vi "Write Hardware Handles.vi"(8 "error in":errorcluster, 10 "hardware handles":T1, 11 "Shared Resources in":refnum<class "Shared Resources.lvclass">) -> (0 "error out":errorcluster, 3 "Shared Resources out":refnum<class "Shared Resources.lvclass">)   [LabVIEW 2020, in "Ballard MIL-STD-1553 Engine.lvlib" / "Implementation.lvlib" / "Shared Resources.lvclass"]
uses:
  Shared Resources.lvclass
  Custom Device/Hardware Handles.ctl
  Shared Resources.lvclass/Shared Resources.ctl
  Custom Device/Custom Device.lvlib
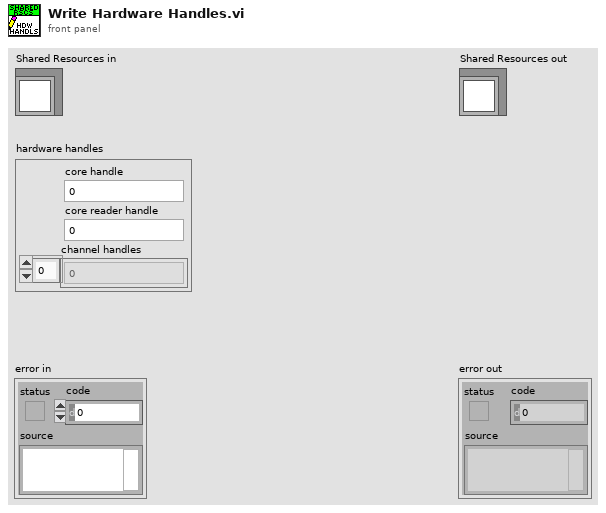
[diagram p1: front panel]
types:
  T1 = typedef "Ballard MIL-STD-1553 Engine.lvlib/Custom Device.lvlib/Hardware Handles.ctl" = cluster{"core handle":u64, "core reader handle":u64, "channel handles":u64[]}
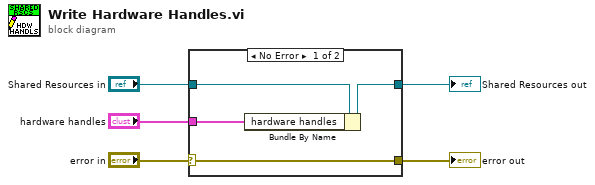
[diagram p0: block diagram]
diagram:
  n1 = case shown="No Error" "error in" {
    selector: "error in" -> [w9 w10]
    tunnel: [w9 w10] -> w4
    tunnel: [w7 w11] -> w2
    tunnel: "Shared Resources in" -> [w8 w11]
    tunnel: "hardware handles" -> [w6 _]
    frame No Error {
      n2 = Bundle By Name(cluster=w8, "hardware handles"=w6) -> (w7:refnum<class "Shared Resources.lvclass">)
    }
    frame Error {
    }
  }
  "error out" <- w4
  "Shared Resources out" <- w2
